vi "ELVIS III Global.vi"() -> ()   [LabVIEW 2019]
panel:
  in  "Timer.IRQ_NO":u8
  in  "SPI.A.IRQ_NO":u8=27
  in  "DO.B.DMA_IRQ_NO":u8=28
  in  "DO.A.DMA_IRQ_NO":u8=29
  in  "AO.B.DMA_IRQ_NO":u8=30
  in  "AO.A.DMA_IRQ_NO":u8=31
  in  "SPI.B.IRQ_NO":u8=26
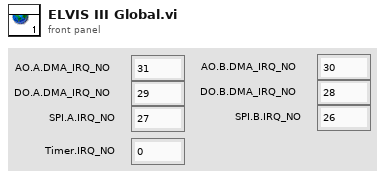
[diagram p1: front panel]
diagram:
